vi "Is Slipping.vi"(11 "Updated Drive Metrics":T1) -> (3 "output cluster":T1)   [LabVIEW 2014]
uses:
  Drive Train Metrics.ctl
  CmdFlag.ctl
  encoderData.vi
  DriveCals.vi
panel:
  out "time of lat slip":u32
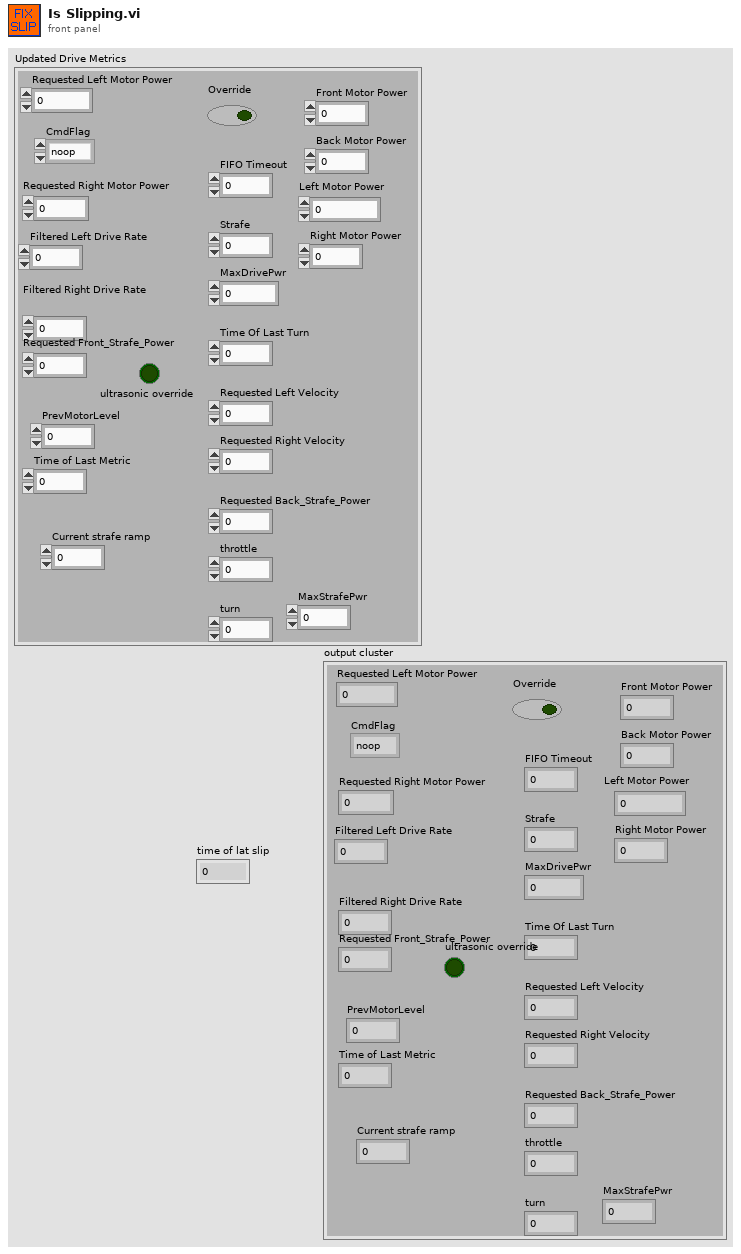
[diagram p1: front panel]
types:
  T1 = typedef "Drive Train Metrics.ctl" = cluster{"CmdFlag":T2, "Requested Right Motor Power":dbl, "Requested Left Motor Power":dbl, "Filtered Left Drive Rate":dbl, "Filtered Right Drive Rate":dbl, "Time of Last Metric":u32, "FIFO Timeout":i32, "Requested Left Velocity":dbl, "Requested Right Velocity":dbl, "throttle":dbl, "turn":dbl, "MaxDrivePwr":dbl, "Strafe":dbl, "Override":bool, "Time Of Last Turn":dbl, "Requested Front_Strafe_Power":dbl, "Requested Back_Strafe_Power":dbl, "MaxStrafePwr":dbl, "PrevMotorLevel":u8, "ultrasonic override":bool, "Left Motor Power":dbl, "Right Motor Power":dbl, "Front Motor Power":dbl, "Back Motor Power":dbl, "Current strafe ramp":dbl}
  T2 = typedef "CmdFlag.ctl" = enum16{"noop", "logflag", "suspend", "resume"}
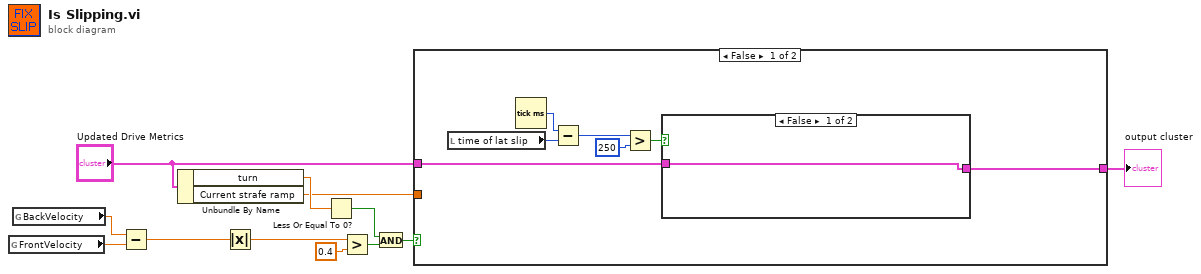
[diagram p0: block diagram]
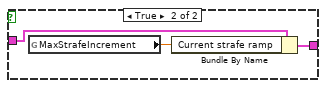
[diagram p2: hidden frame]
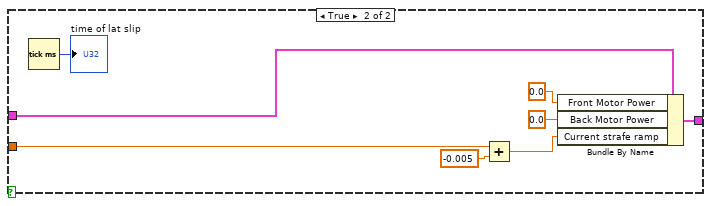
[diagram p3: hidden frame]
diagram:
  n1 = global read "encoderData.vi" "FrontVelocity"() -> (w7:dbl)
  n2 = global read "encoderData.vi" "BackVelocity"() -> (w6:dbl)
  n3 = Subtract(x=w6, y=w7) -> (x-y=w8:dbl)
  n4 = Unbundle By Name("Updated Drive Metrics") -> ("turn"=w5:dbl, "Current strafe ramp"=w1:dbl)
  n5 = Absolute Value(x=w8) -> (abs(x)=w9:dbl)
  n6 = Less Or Equal To 0?(x=w5) -> (x <= 0?=w12:bool)
  n7 = Greater?(x=w9, y=0.4) -> (0:w11:bool)
  n8 = And(x=w12, y=w11) -> (x .and. y?=w4:bool)
  n9 = case shown="False" w4 {
    tunnel: "Updated Drive Metrics" -> [w19 w31]
    tunnel: [w18 w30] -> w2
    tunnel: w1 -> [_ w26]
    frame False {
      n10 = local read "time of lat slip"() -> (w16:u32)
      n11 = Tick Count (ms)() -> (millisecond timer value=w17:u32)
      n12 = Subtract(x=w17, y=w16) -> (x-y=w15:u32)
      n13 = Greater?(x=w15, y=u32 250) -> (0:w13:bool)
      n14 = case shown="False" w13 {
        tunnel: w19 -> [w20 w23]
        tunnel: [w20 w22] -> w18
        frame False {
        }
        frame True {
          n15 = global read "DriveCals.vi" "MaxStrafeIncrement"() -> (w21:dbl)
          n16 = Bundle By Name(cluster=w23, "Current strafe ramp"=w21) -> (w22:T1)
        }
      }
    }
    frame True {
      n17 = Tick Count (ms)() -> (millisecond timer value=→"time of lat slip":u32)
      n18 = Add(x=w26, y=-0.005) -> (x+y=w27:dbl)
      n19 = Bundle By Name(cluster=w31, "Front Motor Power"=0.0, "Back Motor Power"=0.0, "Current strafe ramp"=w27) -> (w30:T1)
    }
  }
  "output cluster" <- w2
